vi "Write Multiple Registers.vi"(8 "error in":errorcluster, 9 "register values":u16[](array[numeric]), 10 "starting address":u16, 11 "Master CR in":refnum<class "WebSocket Client CR.lvclass">) -> (0 "error out":errorcluster, 3 "Master CR out":refnum<class "WebSocket Client CR.lvclass">)   [LabVIEW 2021]
doc: "Writes the values of multiple holding register values in series, starting at address M."
uses:
  WebSocket Client CR.lvclass
  WebSocket Client CR.lvclass/WebSocket Client CR.ctl
  Modbus_v121c/Data Model/Device Data Model.lvclass
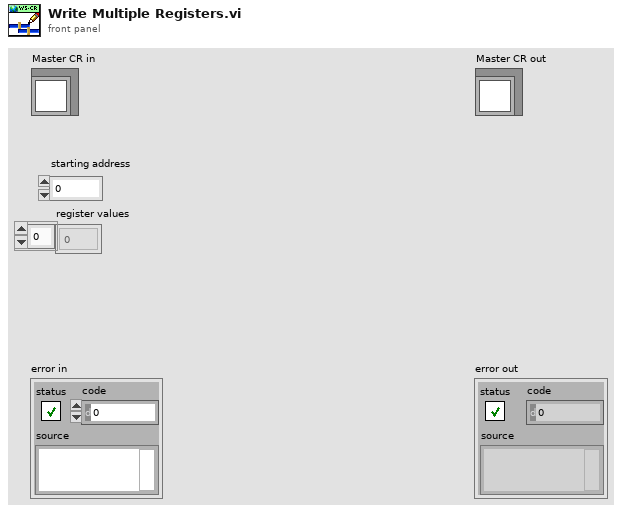
[diagram p1: front panel]
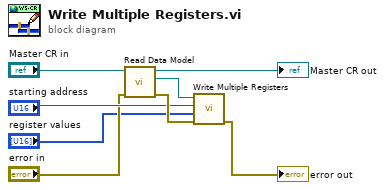
[diagram p0: block diagram]
diagram:
  n1 = call "Read Data Model.vi"("error in (no error)"="error in", "Master CR in"="Master CR in") -> ("error out"=w5:errorcluster, "Data Model"=w6:refnum<class "Device Data Model.lvclass">, "Master CR out"=→"Master CR out":refnum<class "WebSocket Client CR.lvclass">)  [unwired: 7 in]
  n2 = call-dynamic "Write Multiple Registers.vi"("error in"=w5, "register values"="register values", "starting address"="starting address", "device data model in"=w6) -> ("error out"=→"error out":errorcluster)  [unwired: 6 in, 1 out]
